vi "waveform.vi"() -> ()   [LabVIEW 2021]
panel:
  out "Waveform Graph 2":waveform(dbl)(graph)
  out "output waveform":waveform(dbl)
  out "Waveform Graph":waveform(dbl)(graph)
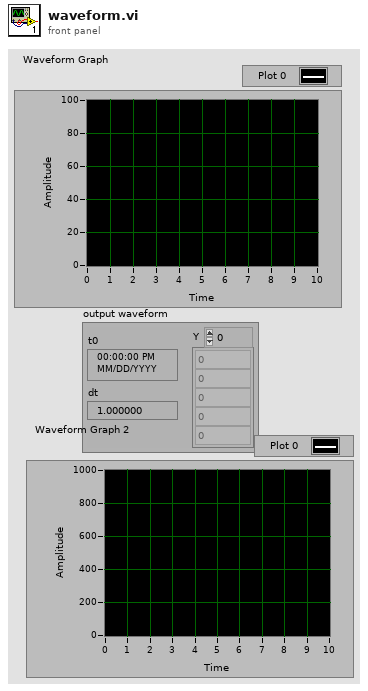
[diagram p1: front panel]
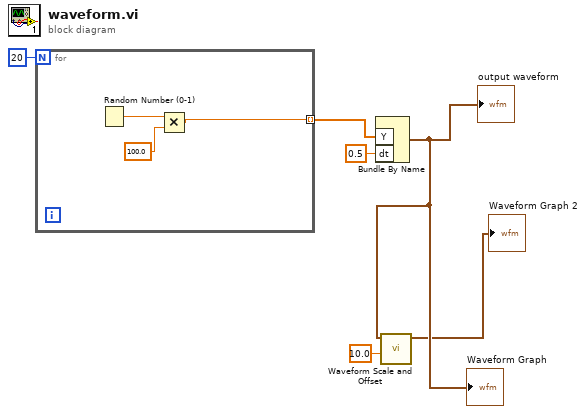
[diagram p0: block diagram]
diagram:
  n1 = for {
    N: 20 -> [_]
    tunnel: [w7] -> w5 mode=indexing
    n2 = Random Number (0-1)() -> (number: 0 to 1=w9:dbl)
    n3 = Multiply(x=w9, y=100.0) -> (x*y=w7:dbl)
  }
  n4 = Bundle By Name("Y"=w5, "dt"=0.5) -> (w3:waveform(dbl))  [unwired: 1 in]
  "Waveform Graph" <- w3
  "output waveform" <- w3
  n5 = call <vilib>:"Waveform Scale and Offset.vi"("scale"=10.0, "waveform in"=w3) -> ("waveform out"=→"Waveform Graph 2":waveform(dbl))  [unwired: 8 in, 1 out]
